vi "Queue_driver.vi"(0 "Array Elements":string[](array[string]), 5 "Element in":string, 11 "error in (no error)":errorcluster, 13 "Operations":T1) -> (4 "Element out":string, 15 "error out":errorcluster)   [LabVIEW 2023, in "Queue_Driver.lvlib"]
doc: "Used to store and perform the queue relaed operations"
uses:
  Queue_Driver.lvlib
  Controls/Queue Opertaions.ctl
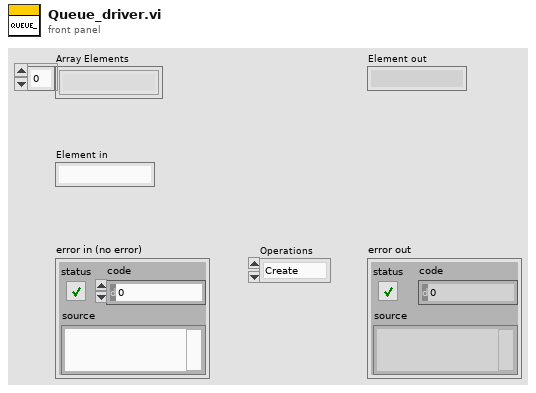
[diagram p1: front panel]
types:
  T1 = typedef "Queue_Driver.lvlib/Queue Opertaions.ctl" = enum16{"Create", "Enqueue", "Enqueue N", "Flush", "Dequeue", "Destroy"}
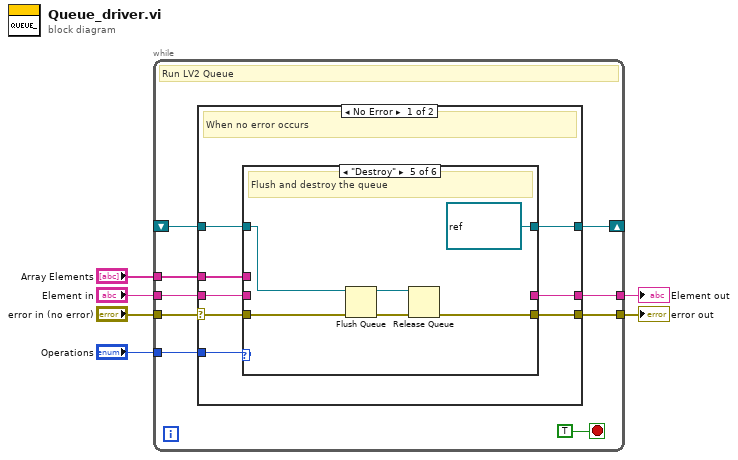
[diagram p0: block diagram]
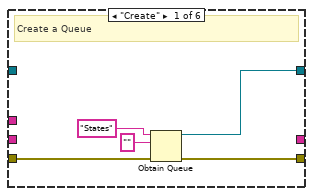
[diagram p2: hidden frame]
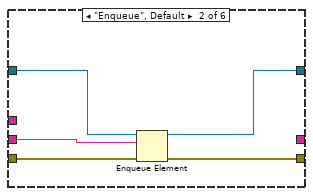
[diagram p3: hidden frame]
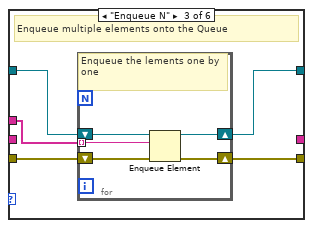
[diagram p4: hidden frame]
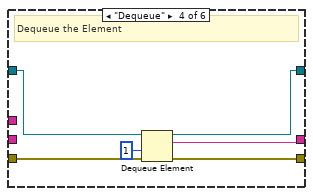
[diagram p5: hidden frame]
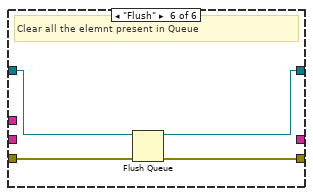
[diagram p6: hidden frame]
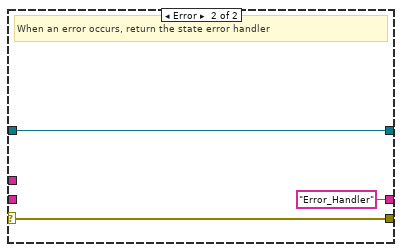
[diagram p7: hidden frame]
diagram:
  n1 = while {
    tunnel: "error in (no error)" -> [w15]
    tunnel: "Operations" -> [w14]
    tunnel: [w13] -> w4
    shift-right: [w12] -> _
    shift-left: _ -> [w11]
    tunnel: "Element in" -> [w10]
    tunnel: "Array Elements" -> [w9]
    tunnel: [w8] -> w1
    stop <- TRUE stop-if-true
    # "Run LV2 Queue"
    n2 = case shown="No Error" w15 {
      selector: w15 -> [w23 w62]
      tunnel: w14 -> [w22 _]
      tunnel: [w21 w62] -> w13
      tunnel: [w20 w61] -> w12
      tunnel: w11 -> [w19 w61]
      tunnel: w10 -> [w18 _]
      tunnel: w9 -> [w17 _]
      tunnel: [w16 "Error_Handler"] -> w8
      frame No Error {
        # "When no error occurs"
        n3 = case shown="\"Destroy\"" w22 {
          tunnel: w23 -> [w26 w33 w38 w49 w55 w59]
          tunnel: [w25 w32 w37 w48 w53 w58] -> w21
          tunnel: [w24 w29 w34 w46 refnum<queue> refnum ("queue out") w56] -> w20
          tunnel: w19 -> [_ w31 w35 w47 w52 w57]
          tunnel: w18 -> [_ w30 _ _ _ _]
          tunnel: w17 -> [_ _ w36 _ _ _]
          tunnel: [_ _ _ w45 _ _] -> w16
          frame "Create" {
            # "Create a Queue"
            n4 = Obtain Queue(name (unnamed)="States", element data type="", error in (no error)=w26) -> (queue out=w24:refnum<queue>, error out=w25:errorcluster)  [unwired: 2 in, 1 out]
          }
          frame "Enqueue", Default {
            n5 = Enqueue Element(queue=w31, element=w30, error in (no error)=w33) -> (queue out=w29:refnum<queue>, error out=w32:errorcluster)  [unwired: 1 in, 1 out]
          }
          frame "Enqueue N" {
            # "Enqueue multiple elements onto the Queue"
            n6 = for {
              shift-right: [w42] -> w37
              shift-left: w38 -> [w43]
              tunnel: w36 -> [w41] mode=indexing
              shift-right: [w39] -> w34
              shift-left: w35 -> [w40]
              # "Enqueue the lements one by one"
              n7 = Enqueue Element(queue=w40, element=w41, error in (no error)=w43) -> (queue out=w39:refnum<queue>, error out=w42:errorcluster)  [unwired: 1 in, 1 out]
            }
          }
          frame "Dequeue" {
            # "Dequeue the Element"
            n8 = Dequeue Element(queue=w47, timeout in ms (-1)=1, error in (no error)=w49) -> (queue out=w46:refnum<queue>, element=w45:string, error out=w48:errorcluster)  [unwired: 1 out]
          }
          frame "Destroy" {
            # "Flush and destroy the queue"
            n9 = Flush Queue(queue=w52, error in (no error)=w55) -> (queue out=w51:refnum<queue>, error out=w54:errorcluster)  [unwired: 1 out]
            n10 = Release Queue(queue=w51, error in (no error)=w54) -> (error out=w53:errorcluster)  [unwired: 1 in, 2 out]
          }
          frame "Flush" {
            # "Clear all the elemnt present in Queue"
            n11 = Flush Queue(queue=w57, error in (no error)=w59) -> (queue out=w56:refnum<queue>, error out=w58:errorcluster)  [unwired: 1 out]
          }
        }
      }
      frame Error {
        # "When an error occurs, return the state error handler"
      }
    }
  }
  "error out" <- w4
  "Element out" <- w1
